vi "sawtooth.vi"() -> ()   [LabVIEW 2025]
uses:
  <vilib>/express/express analysis/Spectral/Block/exnSpectralBlock spectral measurements peak poly.vi
  <vilib>/express/express analysis/Spectral/Block/exnSpectralBlock spectral measurements peak DDT.vi
  <vilib>/express/express analysis/Spectral/XNode/ExpressSpectralMeasurementsBlockNode.xnode
panel:
  out "Waveform Graph 2":dynamicdata(graph)
  out "Waveform Graph":dynamicdata(graph)
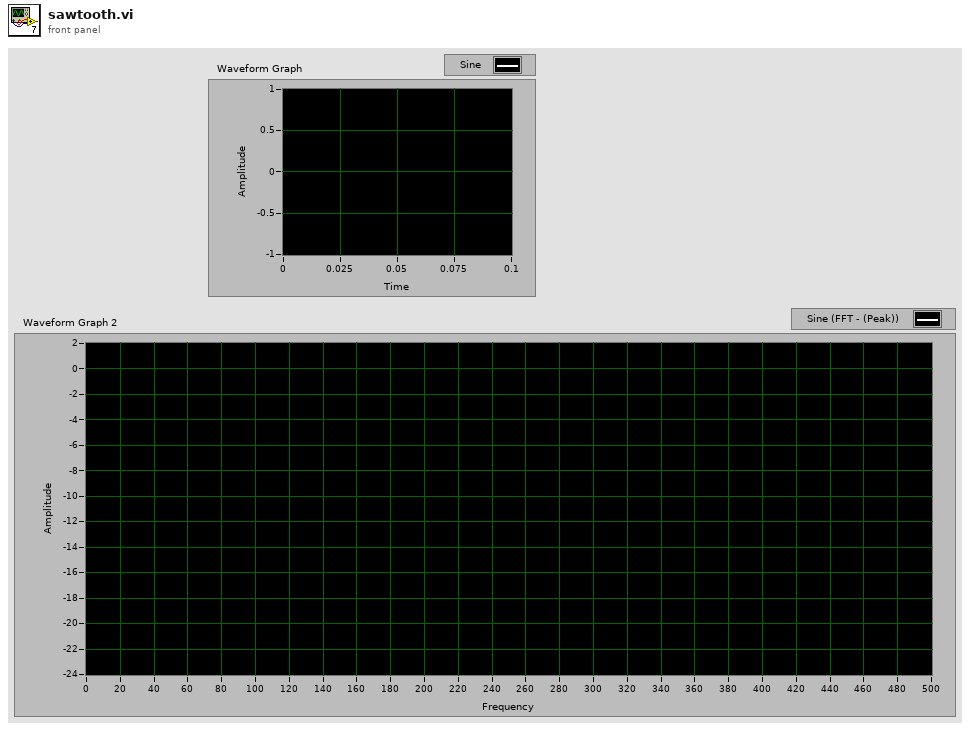
[diagram p1: front panel]
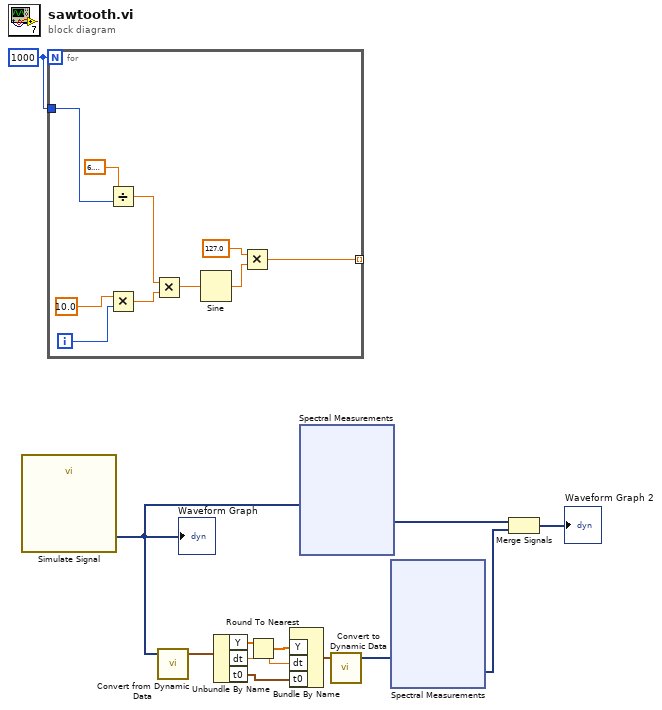
[diagram p0: block diagram]
diagram:
  w12 = 1000
  n1 = call "Simulate Signal"() -> ("Sine"=w9:dynamicdata)  [unwired: 14 in, 1 out]
  "Waveform Graph" <- w9
  n2 = for {
    N: w12 -> [_]
    tunnel: w12 -> [w21]
    tunnel: [w13] -> _ mode=indexing
    i -> [w19]
    n3 = Divide(x=6.283185307179586, y=w21) -> (x/y=w14:dbl)
    n4 = Multiply(x=10.0 ("y"), y=w19) -> (x*y=w15:dbl)
    n5 = Multiply(x=w14, y=w15) -> (x*y=w16:dbl)
    n6 = Sine(x=w16) -> (sin(x)=w17:dbl)
    n7 = Multiply(x=127.0, y=w17) -> (x*y=w13:dbl)
  }
  n8 = call "Convert from Dynamic Data"("Dynamic Data Type"=w9) -> ("Waveform"=w8:waveform(dbl))  [unwired: 3 in]
  n9 = Unbundle By Name(w8) -> ("Y"=w7:dbl[], "dt"=w6:dbl, "t0"=w5:timestamp)
  n10 = Round To Nearest(number=w7) -> (nearest integer value=w1:dbl[])
  n11 = Bundle By Name("Y"=w1, "dt"=w6, "t0"=w5) -> (w4:waveform(dbl))  [unwired: 1 in]
  n12 = xnode "Spectral Measurements"("Signals"=w9) -> ("FFT - (Peak)"=w10:dynamicdata)  [unwired: 1 in, 2 out]
  n13 = call "Convert to Dynamic Data"("Waveform"=w4) -> ("Dynamic Data Type"=w3:dynamicdata)  [unwired: 3 in]
  n14 = xnode "Spectral Measurements"("Signals"=w3) -> ("FFT - (Peak)"=w2:dynamicdata)  [unwired: 1 in, 2 out]
  n15 = Merge Signals(w10, w2) -> (→"Waveform Graph 2":dynamicdata)
